vi "Read EIP tags.vi"(8 "error in":errorcluster, 11 "EIP Tags Configuration in":refnum<class "EIP Tags Configuration.lvclass">) -> (0 "error out":errorcluster, 2 "EIP tags":T1[](array[typedef]), 3 "EIP Tags Configuration out":refnum<class "EIP Tags Configuration.lvclass">)   [LabVIEW 2013, in "EIP Tags Configuration.lvclass"]
uses:
  EIP Tags Configuration.lvclass
  eip tag definition.ctl
  eip tag types.ctl
  EIP Tags Configuration.lvclass/EIP Tags Configuration.ctl
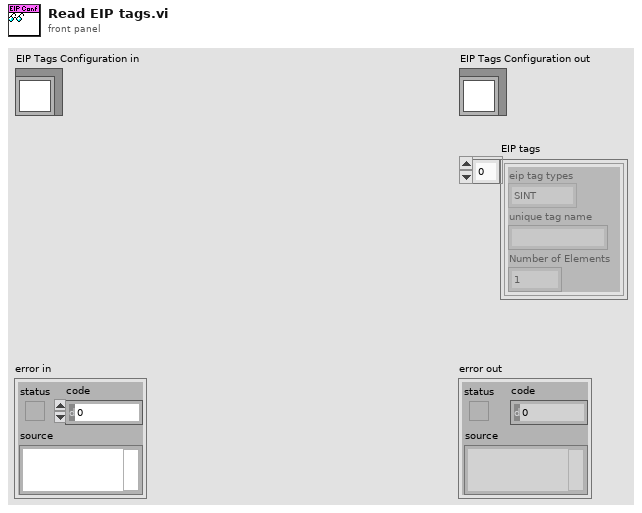
[diagram p1: front panel]
types:
  T1 = typedef "EIP Tags Configuration.lvclass/eip tag definition.ctl" = cluster{"eip tag types":T2, "unique tag name":string, "Number of Elements":u32}
  T2 = typedef "EIP Tags Configuration.lvclass/eip tag types.ctl" = enum16{"SINT", "INT", "DINT", "REAL", "BOOL", "STRING"}
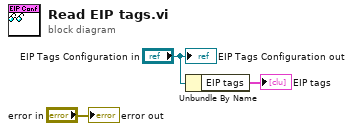
[diagram p0: block diagram]
diagram:
  n1 = Unbundle By Name("EIP Tags Configuration in") -> ("EIP tags"=→"EIP tags":T1[])
  "error out" <- "error in"
  "EIP Tags Configuration out" <- "EIP Tags Configuration in"
